vi "ModuleManager.vi"(10 "Parameters":variant, 11 "Process":refnum<class "Process.lvclass">) -> ()   [LabVIEW 2023, in "Vires VTD Engine.lvlib"]
uses:
  Vires VTD Engine.lvlib
  <vilib>/NI/NIVS Inline Async API/_VS Inline Async API/Process/Process.lvclass
  Shared/Compiled.Settings.ctl
  System Explorer/RDB Data.ctl
  RDB/RDB Object.ctl
  RDB/RDB Player Object.ctl
  Shared/Network Settings.ctl
  Shared/Protocol.ctl
  Shared/SensorInfos.ctl
  Shared/SensorInfo.ctl
  Shared/Sensor Name.ctl
  MM/MM Data.ctl
  MM/MM Objects.ctl
  MM/MM Object.ctl
  Shared/Timedloop Settings.ctl
  <vilib>/NI/NIVS Inline Async API/_VS Inline Async API/Process/Process.lvclass/Process.ctl
  <vilib>/Platform/TimedLoop/XDataNode/timing_clust.ctl
  <vilib>/Platform/TimedLoop/XDataNode/nitl_modes.ctl
  <vilib>/Platform/TimedLoop/XDataNode/wakeup.ctl
  <vilib>/NI/NIVS Inline Async API/_Data Access Engine/Access Type Classes/Write/Write.lvclass/Write.ctl
  <vilib>/NI/NIVS Inline Async API/_Data Access Engine/Data Access Engine/Methods/Write.Data.vi
  <vilib>/NI/NIVS Inline Async API/_VS Inline Async API/Process/Data Member Access/Read Data Access.vi
  <vilib>/NI/NIVS Inline Async API/_VS Inline Async API/Error Handling Process/SubVIs/Error.ConvertArray.vi
  <vilib>/NI/NIVS Inline Async API/_Data Access Engine/Access Type Classes/Write/Write.ProcessData.vi
  <vilib>/NI/NIVS Inline Async API/_Data Access Engine/Access Type Classes/Write/Write.Buffer.vi
  <vilib>/NI/NIVS Inline Async API/_Data Access Engine/Access Type Classes/Write/Write.Commit.vi
  <vilib>/NI/NIVS Inline Async API/_Data Access Engine/Data Access Engine/Methods/Write.Lookup.vi
  <vilib>/NI/NIVS Inline Async API/_Data Access Engine/Data Access Engine/Data Access Engine.lvclass
  <vilib>/platform/TimedLoop/XDataNode/XDataNode.xnode
  Shared/Vires VTD Shared.lvlib
  RDB/RDB.lvlib
  MM/MM.lvlib
  <vilib>/Platform/TimedLoop/XDataNode/XDNodeRunTimeDep.lvlib
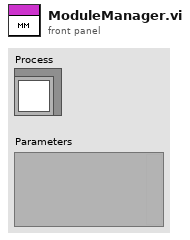
[diagram p1: front panel]
types:
  T1 = typedef "Vires VTD Shared.lvlib/Compiled.Settings.ctl" = cluster{"Name":string, "RDB Data Receive ":T2, "RDB Data Sent":T2, "vclient":path, "Network Settings":T5, "SensorInfos":T7, "mmanager":path, "Scenario Paths":string[], "Custom SCP Commands":string[], "Timed Loop Settings for TaskControl":T13, "Timed Loop Settings for ModuleManager":T13}
  T2 = typedef "Vires VTD Shared.lvlib/RDB Data.ctl" = T3[]
  T3 = typedef "RDB.lvlib/RDB Object.ctl" = cluster{"pkID":i32, "RDB Player Objects":T4[]}
  T4 = typedef "RDB.lvlib/RDB Player Object.ctl" = cluster{"PlayerID":i32, "Signals":string[], "adv para":i32}
  T5 = typedef "Vires VTD Shared.lvlib/Network Settings.ctl" = cluster{"IP adress":string, "RDB":cluster{"Protocol":T6, "Tx Port":u16, "Rx Port":u16, "Buffer Size":i32, "Timeout":u16}, "SCP":cluster{"Protocol":T6, "Tx Port":u16, "Rx Port":u16, "Buffer Size":i32, "Timeout":u16}}
  T6 = typedef "Vires VTD Shared.lvlib/Protocol.ctl" = enum16{"UDP", "TCP"}
  T7 = typedef "Vires VTD Shared.lvlib/SensorInfos.ctl" = T8[]
  T8 = typedef "Vires VTD Shared.lvlib/SensorInfo.ctl" = cluster{"Sensor Name":T9, "Protocol":T6, "Network port":i32, "# Culled Objects":i32, "PlayerID":u8, "MM Data":T10}
  T9 = typedef "Vires VTD Shared.lvlib/Sensor Name.ctl" = string
  T10 = typedef "Vires VTD Shared.lvlib/MM Data.ctl" = T11[]
  T11 = typedef "MM.lvlib/MM Objects.ctl" = cluster{"pkID":i32, "MM Objects":T12[]}
  T12 = typedef "MM.lvlib/MM Object.ctl" = cluster{"Object":i32, "Signals":string[]}
  T13 = typedef "Vires VTD Shared.lvlib/Timedloop Settings.ctl" = cluster{"Period(ms)":i64, "Priority":i32, "Processor":i32}
  T14 = typedef "Data Access Engine.lvlib/Data Access Engine.lvclass/Write.DVR.ctl" = refnum<data-value>
  T15 = typedef "MM.lvlib/Sensor Engine Data.ctl" = cluster{"TCP Network":refnum<k5>, "UDP Network":refnum<k16>, "Network port":i32, "Protocol":T6, "Sensor Name":T9, "Signal Data":dbl[], "MM Frames":T16[], "MM Culled Objects":i32[], "MM Frame Refs":refnum<k21>[], "mmanager":path}
  T16 = typedef "XNET Frame FlexRay.ctl" = cluster{"timestamp":timestamp, "payload":u8[], "slot":u16, "type":T17, "cycle count":u8, "startup?":bool, "sync?":bool, "preamble?":bool, "ch A":bool, "ch B":bool, "echo?":bool}
  T17 = typedef "XNET Frame Type FlexRay.ctl" = u8
  T18 = typedef "XDNodeRunTimeDep.lvlib/timing_clust.ctl" = cluster{"Expected End [f-1]":u64, "Actual End [f-1]":u64, "Finished Late? [f-1]":bool, "Expected End [i-1]":u64, "Actual End [i-1]":u64, "Finished Late? [i-1]":bool, "Expected Start [i]":u64, "Actual Start [i]":u64, "Expected Start [f]":u64, "Actual Start [f]":u64, "Source Name":string, "Structure Name":string, "Period":i64, "Deadline":i64, "Offset":i64, "Start":i64, "Priority":i32, "Timeout":i32, "Mode":T19, "Wakeup Reason":T20, "Error":errorcluster, "Source Type":string, "Secondary Source Type":string, "Global End Time":u64, "Global Start Time":u64, "Frame Duration":u64, "Iteration Duration":u64, "Assigned CPU":i32, "I/O Scan Engine Mode":u32}
  T19 = typedef "XDNodeRunTimeDep.lvlib/nitl_modes.ctl" = enum32{"No Change", "Process missed periods, maintain original phase", "Discard missed periods, maintain original phase", "Process missed periods, ignore original phase", "Discard missed periods, ignore original phase"}
  T20 = typedef "XDNodeRunTimeDep.lvlib/wakeup.ctl" = enum32{"Normal", "Aborted", "Asynchronous wakeup", "Timing source error", "Timed loop error", "Timeout"}
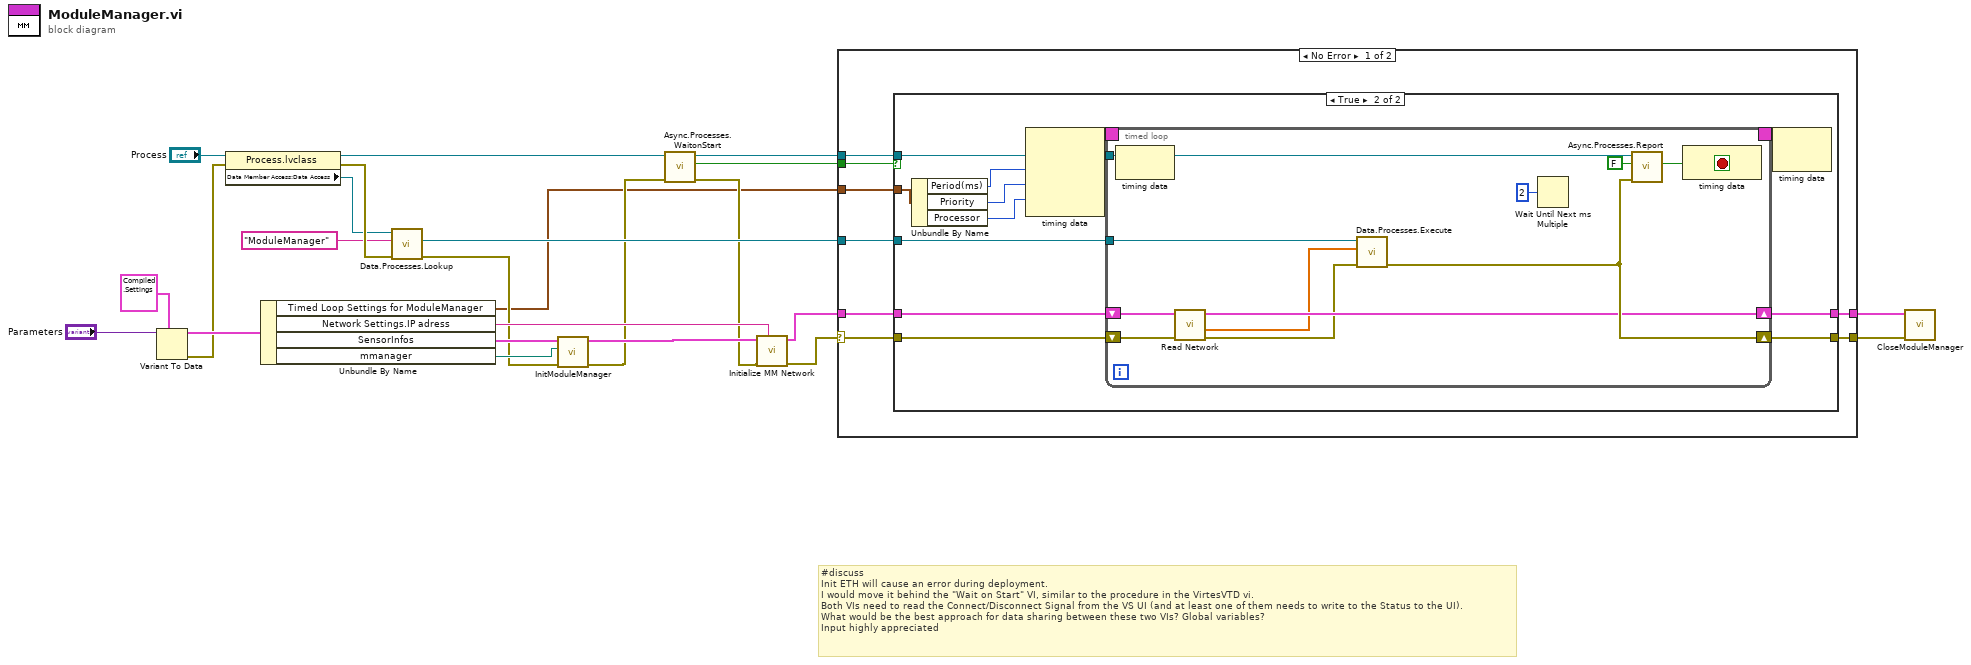
[diagram p0: block diagram]
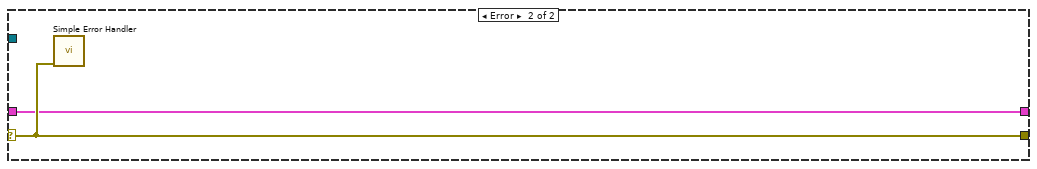
[diagram p3: hidden frame]
diagram:
  # "#discuss\nInit ETH will cause an error during deployment.\nI would move it behind the \"Wait on Start\" VI, similar to the procedure in the VirtesVTD vi.\nBoth VIs need to read the Connect/Disconnect Signal from the VS UI (and at least one of them needs to write to the Status to the UI).\nWhat would be the best approach for data sharing between these two VIs? Global variables?\nInput highly appreciated"
  n1 = Variant To Data(type=T1 {"Name"="", "RDB Data Receive "=[], "RDB Data Sent"=[], "vclient"=path "", "Network Settings"={"IP adress"="127.0.0.1", "RDB"={"Protocol"=enum."TCP", "Tx Port"=10, "Rx Port"=10, "Buffer Size"=204800, "Timeout"=10}, "SCP"={"Protocol"=enum."UDP", "Tx Port"=48190, "Rx Port"=48190, "Buffer Size"=204800, "Timeout"=10}}, "SensorInfos"=[], "mmanager"=path "", "Scenario Paths"=[], "Custom SCP Commands"=[], "Timed Loop Settings for TaskControl"={"Period(ms)"=2, "Priority"=100, "Processor"=-2}, "Timed Loop Settings for ModuleManager"={"Period(ms)"=2, "Priority"=100, "Processor"=-2}} ("Compiled.Settings"), Variant="Parameters") -> (data=w14:T1, error out=w6:errorcluster)  [unwired: 1 in]
  n2 = property class="Process.lvclass"(reference="Process", error in=w6) -> (reference out=w21:refnum<class "Process.lvclass">, error out=w18:errorcluster, "Data Member Access:Data Access"=w17:refnum<class "Data Access Engine.lvclass">)
  n3 = Unbundle By Name(w14) -> ("Timed Loop Settings for ModuleManager"=w1:T13, "Network Settings.IP adress"=w11:string, "SensorInfos"=w10:T7, "mmanager"=w7:path)
  n4 = call-poly <vilib>:"Data.Processes.Lookup.vi"("error in (no error)"=w18, "Name"="ModuleManager" ("Item Name"), "Data Access API in"=w17) -> ("error out"=w5:errorcluster, "Ref"=w15:T14)  [unwired: 5 in, 2 out]
  n5 = call "InitModuleManager.vi"("error in (no error)"=w5, "mmanager"=w7, "SensorInfos"=w10) -> ("error out (no error)"=w4:errorcluster, "Sensor Engine Datas"=w13:T15[])  [unwired: 7 in]
  n6 = call <vilib>:"Async.Processes.WaitonStart.vi"("error in (no error)"=w4, "Process"=w21) -> ("error out"=w3:errorcluster, "Execute"=w24:bool, "Process out"=w23:refnum<class "Process.lvclass">)  [unwired: 7 in]
  n7 = call "Initialize MM Network.vi"("Net Adress"=w11, "error in (no error)"=w3, "Sensor Engine Datas in"=w13) -> ("error out"=w2:errorcluster, "Sensor Engine Datas out"=w12:T15[])  [unwired: 7 in]
  n8 = case shown="No Error" w2 {
    selector: w2 -> [w30 w67]
    tunnel: w24 -> [w32 _]
    tunnel: w23 -> [w31 _]
    tunnel: w15 -> [w29 _]
    tunnel: [w28 w67] -> w9
    tunnel: w12 -> [w27 w66]
    tunnel: [w26 w66] -> w8
    tunnel: w1 -> [w25 _]
    frame No Error {
      n9 = case shown="True" w32 {
        tunnel: w30 -> [w34 w46]
        tunnel: w31 -> [_ w45]
        tunnel: w29 -> [_ w44]
        tunnel: [w34 w43] -> w28
        tunnel: w27 -> [w33 w42]
        tunnel: [w33 w41] -> w26
        tunnel: w25 -> [_ w38]
        frame False {
        }
        frame True {
          n10 = Unbundle By Name(w38) -> ("Period(ms)"=w37:i64, "Priority"=w36:i32, "Processor"=w35:i32)
          n11 = node-c288(w37, w36, w35) -> (w40:T18)  [unwired: 1 in]
          n12 = timed-loop {
            tunnel: w45 -> [w57]
            tunnel: w44 -> [w54]
            shift-right: [w53] -> w43
            shift-left: w46 -> [w52]
            shift-right: [w50] -> w41
            shift-left: w42 -> [w51]
            timing: w40 -> [_]
            timing-out: [_] -> w39
            stop <- w56 stop-if-true
            n13 = node-c288() -> ()  [unwired: 1 in, 1 out]
            n14 = call "Read Network.vi"("error in (no error)"=w52, "Sensor Engine Datas in"=w51) -> ("error out"=w49:errorcluster, "signal data"=w48:dbl[], "Sensor Engine Datas out"=w50:T15[])  [unwired: 7 in]
            n15 = call-poly <vilib>:"Data.Processes.Execute.vi"("error in (no error)"=w49, "Values"=w48, "Ref"=w54) -> ("error out"=w53:errorcluster)  [unwired: 8 in]
            n16 = Wait Until Next ms Multiple(millisecond multiple=u32 2) -> ()  [unwired: 1 out]
            n17 = call <vilib>:"Async.Processes.Report.vi"("Error"=w53, "Stop Async on Error?"=FALSE, "Process in"=w57) -> ("Stop"=w56:bool)  [unwired: 7 in, 1 out]
            n18 = node-c288() -> ()  [unwired: 1 in, 1 out]
          }
          n19 = node-c288(w39) -> ()  [unwired: 1 out]
        }
      }
    }
    frame Error {
      n20 = call <vilib>:"Simple Error Handler.vi"("error in (no error)"=w67) -> ()  [unwired: 4 in, 5 out]
    }
  }
  n21 = call "CloseModuleManager.vi"("error in (no error)"=w9, "Sensor Engine Datas in"=w8) -> ()  [unwired: 8 in, 2 out]
